vi "Remove ATML DataPlugin.vi"(8 "error in":errorcluster, 11 "name":string) -> (0 "error out":errorcluster)   [LabVIEW 2023]
doc: "When run as an executable, this VI takes command line arguments and passes them to the Unregister DataPlugin VI to unregister the specified DataPlugin on the computer running the executable. When run as a VI, it unregisters the DataPlugin specified by name."
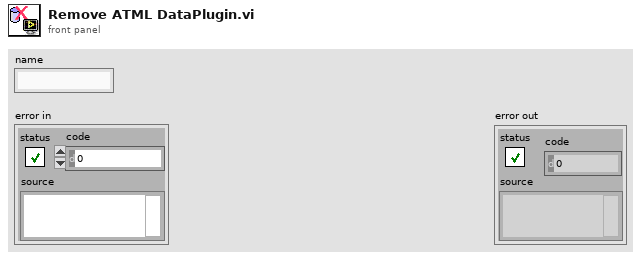
[diagram p1: front panel]
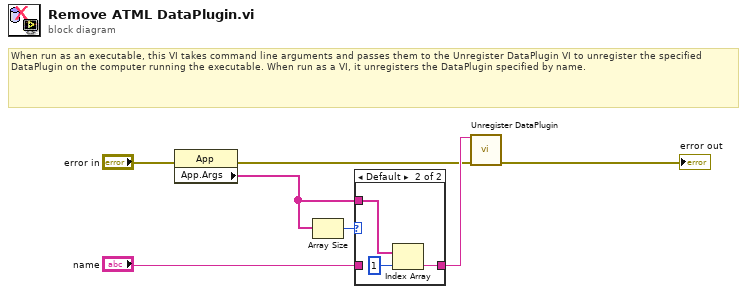
[diagram p0: block diagram]
diagram:
  # "When run as an executable, this VI takes command line arguments and passes them to the Unregister DataPlugin VI to unregister the specified DataPlugin on the computer running the executable. When run as a VI, it unregisters the DataPlugin specified by name."
  n1 = property class="App"(error in="error in") -> (error out=w1:errorcluster, "App.Args"=w6:string[])  [unwired: 1 in, 1 out]
  n2 = Array Size(array=w6) -> (size(s)=w5:i32)
  n3 = case shown="Default" w5 {
    tunnel: "name" -> [w8 _]
    tunnel: w6 -> [_ w11]
    tunnel: [w8 w10] -> w7
    frame 1 {
    }
    frame Default {
      n4 = Index Array(array=w11, index=1) -> (element=w10:string)
    }
  }
  n5 = call <vilib>:"Unregister DataPlugin.vi"("DataPlugin name"=w7, "error in (no error)"=w1) -> ("error out"=→"error out":errorcluster)  [unwired: 13 in]
